vi "NoteEdge_Create.vi"(0 "reference":refnum<class "NoteEdge.lvclass">, 5 "error in (no error)":errorcluster) -> (14 "reference out":refnum<class "NoteEdge.lvclass">, 19 "error out":errorcluster)   [LabVIEW 2012, in "NoteEdge.lvclass"]
doc: "Creates and initializes a new NoteEdge object.\n\nThis object should be destroyed using a NoteEdge destructor VI or a virtual base class destructor VI.\n\n[GOOP 2.1]"
uses:
  <resource>/Framework/Providers/Open_GDS/UML/NoteEdge_class/NoteEdge.lvclass
  <resource>/Framework/Providers/Open_GDS/UML/GeneralPathEdge_class/GeneralPathEdge.lvclass
panel:
  # "The input reference should only\nbe wired when this method is called\nby a sub class constructor."
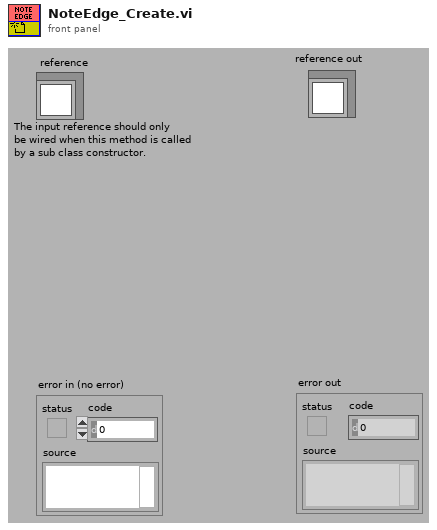
[diagram p1: front panel]
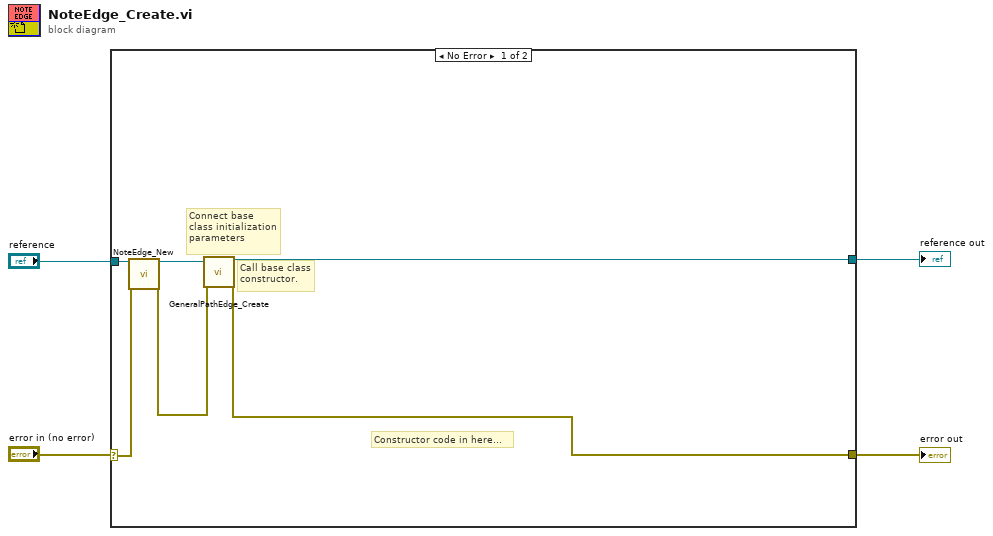
[diagram p0: block diagram]
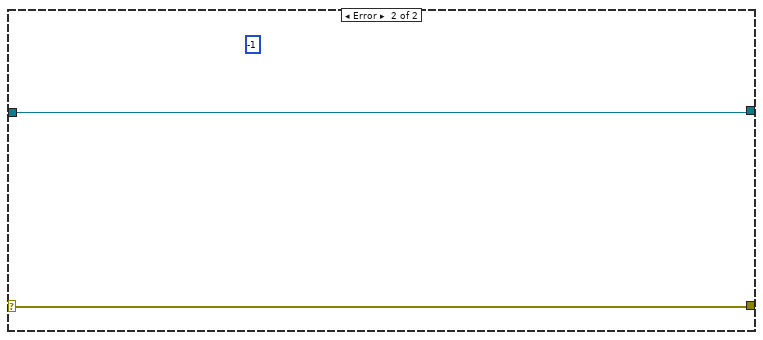
[diagram p2: hidden frame]
diagram:
  n1 = case shown="No Error" "error in (no error)" {
    selector: "error in (no error)" -> [w10 w12]
    tunnel: [w6 w11] -> w4
    tunnel: [w5 w12] -> w3
    tunnel: "reference" -> [w9 w11]
    frame No Error {
      # "Connect base\nclass initialization\nparameters"
      # "Constructor code in here..."
      # "Call base class\nconstructor."
      n2 = call <resource>:"NoteEdge_New.vi"("reference in"=w9, "error in (no error)"=w10) -> ("reference out"=w7:refnum<class "NoteEdge.lvclass">, "error out"=w8:errorcluster)  [unwired: 2 in, 14 out]
      n3 = call <resource>:"GeneralPathEdge_Create.vi"("reference"=w7, "error in (no error)"=w8) -> ("reference out"=w6:refnum<class "NoteEdge.lvclass">, "error out"=w5:errorcluster)  [unwired: 1 in, 15 out]
    }
    frame Error {
      (unwired) -1 ("Nr of open handles")
    }
  }
  "error out" <- w3
  "reference out" <- w4
